vi "XIPIN_Video_Timing_Controller_2_1.vi"   [LabVIEW 2017]
doc: "The Xilinx Video Timing Controller LogiCORE(TM) is a general purpose video timing generator and detector. Automatic detection of horizontal and vertical front and back porches, sync pulses and active video pixels is provided along with sync and blank pulse polarity detection. Horizontal and vertical blanking and sync pulses are generated including support for programmable pulse polarity. The core is programmable through a comprehensive register set allowing control of various timing generation parameters including horizontal and vertical front and back porch start, active video start, sync start and more. A comprehensive set of interrupt status bits is provided for processor monitoring.\n------------------------------------\n<b>Need License</b> : Yes"
uses:
  <vilib>/rvi/XilinxIP/XIPIN_XNode/niFpgaXIPIN.xnode
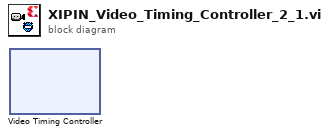
[diagram p0: block diagram]
diagram:
  n1 = xnode ("Video Timing Controller")() -> ()
